vi "PathPlanner_PathFinder_IsCollision.vi"(9 "sEnd":T1, 11 "sStartLoc":T1) -> (3 "Collision":bool)   [LabVIEW 2019]
uses:
  PathPlannerLib24/TypeDef/PathPlannerFinderGridPosition.ctl
  PathPlannerLib24/VI/PathPlanner_PathFinder_Globals.vi
  PathPlannerLib24/PathPlanner24.lvlib
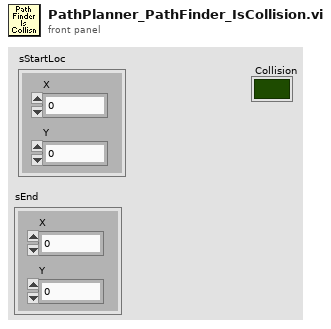
[diagram p1: front panel]
types:
  T1 = typedef "PathPlanner24.lvlib/PathPlannerFinderGridPosition.ctl" = cluster{"X":i32, "Y":i32}
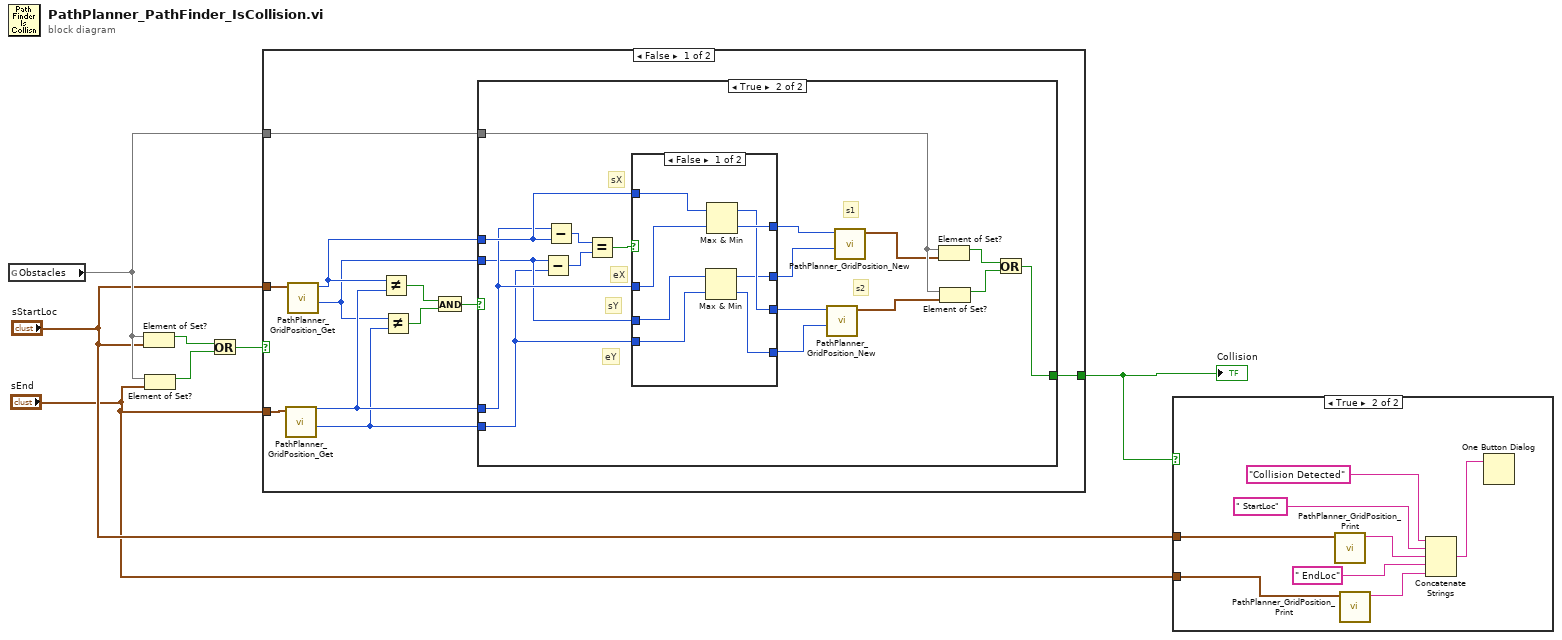
[diagram p0: block diagram]
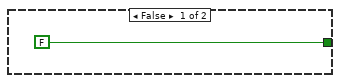
[diagram p3: hidden frame]
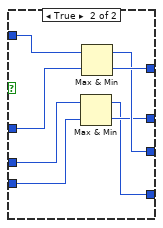
[diagram p4: hidden frame]
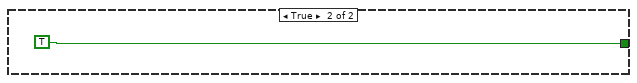
[diagram p5: hidden frame]
diagram:
  n1 = global read "PathPlanner_PathFinder_Globals.vi" "Obstacles"() -> (w4:set{T1})
  n2 = Element of Set?(10:"sStartLoc", 11:w4) -> (3:w7:bool)
  n3 = Element of Set?(10:"sEnd", 11:w4) -> (3:w6:bool)
  n4 = Or(x=w7, y=w6) -> (x .or. y?=w5:bool)
  n5 = case shown="False" w5 {
    tunnel: [w13 TRUE ("Collision")] -> w3
    tunnel: "sStartLoc" -> [w18 _]
    tunnel: "sEnd" -> [w17 _]
    tunnel: w4 -> [w8 _]
    frame False {
      n6 = call "PathPlanner_GridPosition_Get.vi"("GridPosition"=w17) -> ("Int Y"=w9:i32, "Int X"=w12:i32)  [unwired: 9 in]
      n7 = call "PathPlanner_GridPosition_Get.vi"("GridPosition"=w18) -> ("Int Y"=w10:i32, "Int X"=w11:i32)  [unwired: 9 in]
      n8 = Not Equal?(x=w11, y=w12) -> (x != y?=w15:bool)
      n9 = Not Equal?(x=w10, y=w9) -> (x != y?=w14:bool)
      n10 = And(x=w15, y=w14) -> (x .and. y?=w16:bool)
      n11 = case shown="True" w16 {
        tunnel: [FALSE w20] -> w13
        tunnel: w12 -> [_ w32]
        tunnel: w11 -> [_ w33]
        tunnel: w10 -> [_ w31]
        tunnel: w9 -> [_ w30]
        tunnel: w8 -> [_ w23]
        frame False {
        }
        frame True {
          # "s2"
          # "s1"
          # "eY"
          # "sY"
          # "eX"
          # "sX"
          n12 = Subtract(x=w31, y=w30) -> (x-y=w35:i32)
          n13 = Subtract(x=w32, y=w33) -> (x-y=w36:i32)
          n14 = Equal?(x=w36, y=w35) -> (x = y?=w34:bool)
          n15 = case shown="False" w34 {
            tunnel: [w42 w52] -> w29
            tunnel: [w38 w46] -> w28
            tunnel: w33 -> [w44 w51]
            tunnel: w32 -> [w43 w50]
            tunnel: [w41 w49] -> w27
            tunnel: w31 -> [w40 w48]
            tunnel: w30 -> [w39 w47]
            tunnel: [w37 w45] -> w26
            frame False {
              n16 = Max & Min(x=w40, y=w39) -> (max(x,y)=w38:i32, min(x,y)=w37:i32)
              n17 = Max & Min(x=w44, y=w43) -> (max(x,y)=w41:i32, min(x,y)=w42:i32)
            }
            frame True {
              n18 = Max & Min(x=w48, y=w47) -> (max(x,y)=w45:i32, min(x,y)=w46:i32)
              n19 = Max & Min(x=w51, y=w50) -> (max(x,y)=w49:i32, min(x,y)=w52:i32)
            }
          }
          n20 = call "PathPlanner_GridPosition_New.vi"("Int Y"=w26, "Int X"=w27) -> ("GridPosition"=w21:T1)  [unwired: 9 in]
          n21 = call "PathPlanner_GridPosition_New.vi"("Int Y"=w28, "Int X"=w29) -> ("GridPosition"=w22:T1)  [unwired: 9 in]
          n22 = Element of Set?(10:w22, 11:w23) -> (3:w25:bool)
          n23 = Element of Set?(10:w21, 11:w23) -> (3:w24:bool)
          n24 = Or(x=w25, y=w24) -> (x .or. y?=w20:bool)
        }
      }
    }
    frame True {
    }
  }
  "Collision" <- w3
  n25 = case shown="True" w3 {
    tunnel: "sStartLoc" -> [_ w61]
    tunnel: "sEnd" -> [_ w60]
    frame False {
    }
    frame True {
      n26 = call "PathPlanner_GridPosition_Print.vi"("GridPosition"=w61) -> ("Position String"=w58:string)  [unwired: 10 in]
      n27 = call "PathPlanner_GridPosition_Print.vi"("GridPosition"=w60) -> ("Position String"=w59:string)  [unwired: 10 in]
      n28 = Concatenate Strings("Collision Detected" ("string"), " StartLoc" ("string"), w58, " EndLoc" ("string"), w59) -> (w54:string)
      n29 = One Button Dialog(message=w54) -> ()  [unwired: 1 in, 1 out]
    }
  }
